vi "Lockin Take Data - Outputs.vi"(8 "error in (no error)":errorcluster caption="Error in (no error)") -> (0 "output2":dbl format="%#_12g", 1 "output1":dbl format="%#_12g", 2 "output2":string, 3 "output1":string, 4 "error out":errorcluster caption="Error")   [LabVIEW 2009, in "SR830.lvlib"]
doc: "Reads the values currently displayed on the front panel of the lock-in detector."
uses:
  Global/GPIB Numbers.vi
  sr830/SR830.lvlib
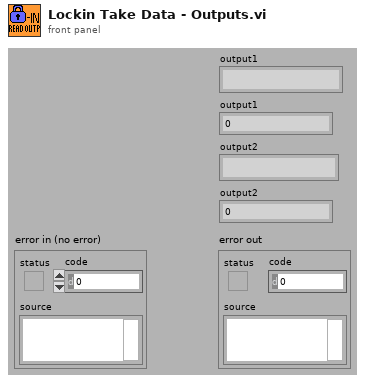
[diagram p1: front panel]
types:
  T1 = typedef "GPIB Type Def.ctl" = cluster{"Name":string, "bus":dbl, "GPIB":dbl, "GPIB as string":string, "byte":i32, "VISA Resource Name":refnum<visa-resource-name>}
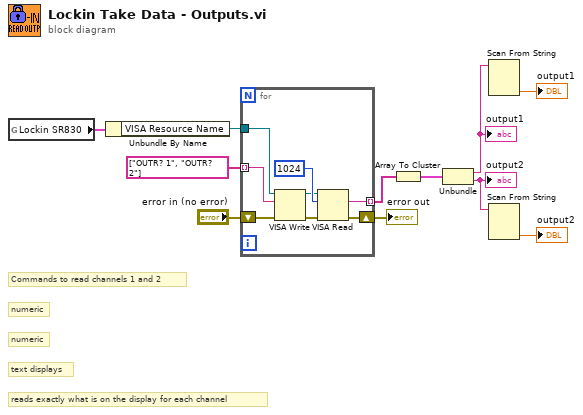
[diagram p0: block diagram]
diagram:
  # "Commands to read channels 1 and 2"
  # "numeric"
  # "numeric"
  # "text displays"
  # "reads exactly what is on the display for each channel"
  n1 = global read "GPIB Numbers.vi" "Lockin SR830"() -> (w3:T1)
  n2 = Unbundle By Name(w3) -> ("VISA Resource Name"=w2:refnum<visa-resource-name>)
  n3 = for {
    tunnel: [w15] -> w8 mode=indexing
    shift-right: [w17] -> w11
    shift-left: "error in (no error)" -> [w16]
    tunnel: w2 -> [w14]
    tunnel: string[] ["OUTR? 1", "OUTR? 2"] -> [w12] mode=indexing
    n4 = VISA Write(VISA resource name=w14, write buffer=w12, error in (no error)=w16) -> (VISA resource name out=w13:refnum<visa-resource-name>, error out=w19:errorcluster)  [unwired: 1 out]
    n5 = VISA Read(VISA resource name=w13, byte count=1024, error in (no error)=w19) -> (read buffer=w15:string, error out=w17:errorcluster)  [unwired: 2 out]
  }
  "error out" <- w11
  n6 = Array To Cluster(array=w8) -> (cluster=w9:cluster{"[0]":string, "[1]":string})
  n7 = Unbundle(w9) -> ("[0]"=w7:string, "[1]"=w6:string)
  "output1" <- w7
  "output2" <- w6
  n8 = Scan From String(input string=w7) -> (output 1=→"output1":dbl)  [unwired: 3 in, 4 out]
  n9 = Scan From String(input string=w6) -> (output 1=→"output2":dbl)  [unwired: 3 in, 4 out]
